vi "AddPackageToCEPMFeed.vi"(8 "Error In":errorcluster, 11 "Package Path":path) -> (0 "Error Out":errorcluster)   [LabVIEW 2019, in "CEPM.lvlib"]
uses:
  CEPM.lvlib
  <vilib>/National Instruments/NIPM API (Beta)/NIPM_API.lvlib
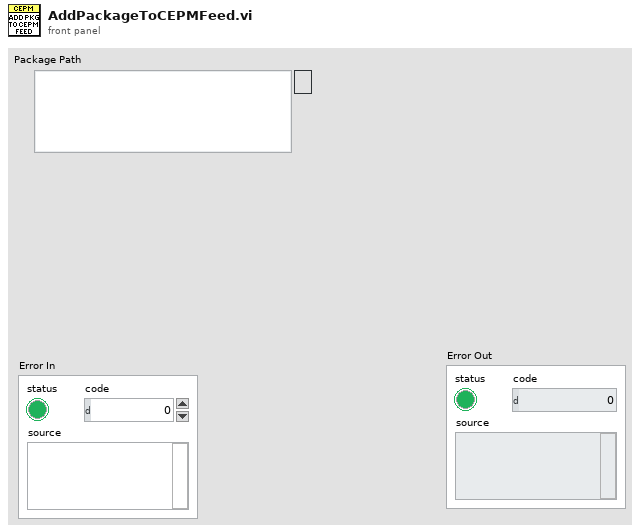
[diagram p1: front panel]
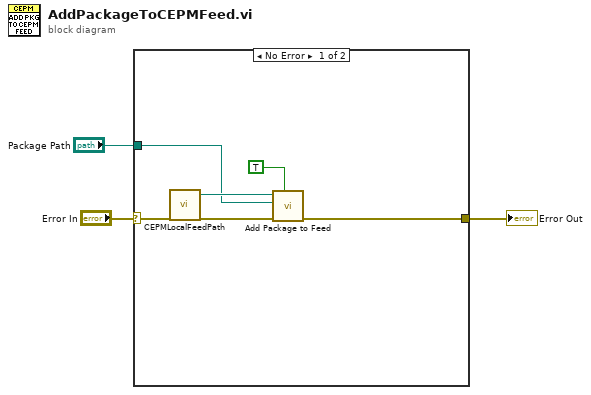
[diagram p0: block diagram]
diagram:
  n1 = case shown="No Error" "Error In" {
    selector: "Error In" -> [w9 w10]
    tunnel: [w4 w10] -> w2
    tunnel: "Package Path" -> [w7 _]
    frame No Error {
      n2 = call "CEPMLocalFeedPath.vi"("Error In"=w9) -> ("Error Out"=w6:errorcluster, "CEPM Local Feed Path"=w8:path)  [unwired: 9 in]
      n3 = call <vilib>:"Add Package to Feed.vi"("create new feed if none exists (F)"=TRUE, "error in"=w6, "package source filepath"=w7, "feed folderpath in"=w8) -> ("error out"=w4:errorcluster)  [unwired: 5 in, 2 out]
    }
    frame Error {
    }
  }
  "Error Out" <- w2
